vi "movearea.vi"(8 "error in (no error)":errorcluster, 11 "Input":string="y-") -> (0 "error out":errorcluster={"status"=TRUE, "code"=56, "source"="LabVIEWSMTPClient.lvlib:Send.vi:2280002<APPEND>\n\n<b>Complete call chain:</b>\r\n     LabVIEWSMTPClient.lvlib:Send.vi:2280002\r\n     Send Email using SMTP Client.vi:2070001\r\n     movearea.vi\r\n     parse and execute command.vi\r\n     TCPIP.Server v2.vi"}, 3 "Output":string="Approach area changed with 0 crashes ")   [LabVIEW 2014]
uses:
  <userlib>/Nanonis Prog Interface V5/Nanonis Prog Interface.lvlib
panel:
  out "num steps z":dbl=500.0
  out "testing?":bool
  out "status":string="approaching"
  in  "STMStatus":T1 {"Size (m)"."Height" format="%.2p"; "Size (m)"."Width" format="%.2p"; "Current (A)" format="%#_6p"; "Z position (m)" format="%#_6p"; "Center coordinates (m)"."Yc" format="%.2p"; "Center coordinates (m)"."Xc" format="%.2p"}
  out "size(s)":i32=1
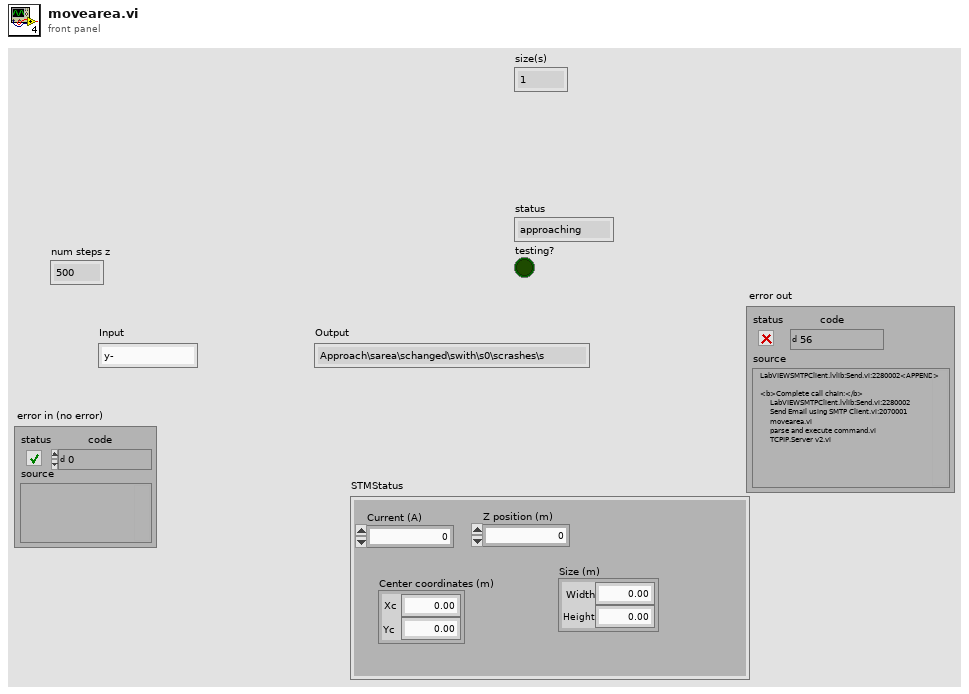
[diagram p1: front panel]
types:
  T1 = cluster{"Center coordinates (m)":cluster{"Xc":sgl, "Yc":sgl}, "Z position (m)":sgl, "Current (A)":sgl, "Size (m)":cluster{"Width":sgl, "Height":sgl}}
  T2 = enum8{"Group 1", "Group 2", "Group 3", "Group 4", "Group 5", "Group 6"}
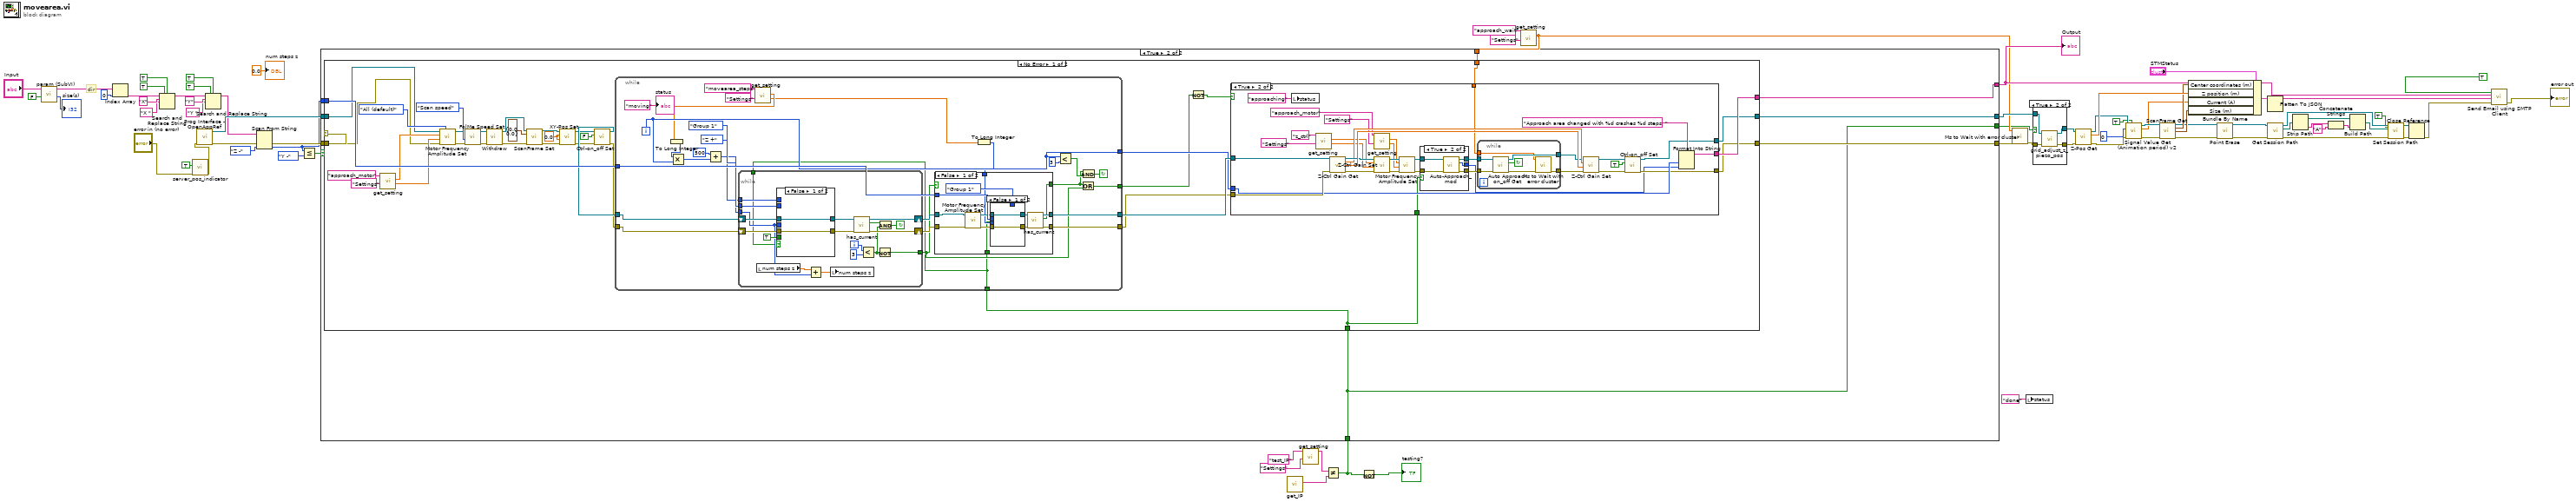
[diagram p0: block diagram]
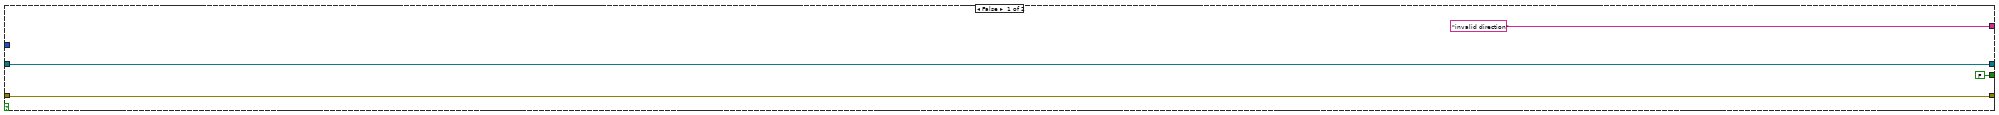
[diagram p3: hidden frame]
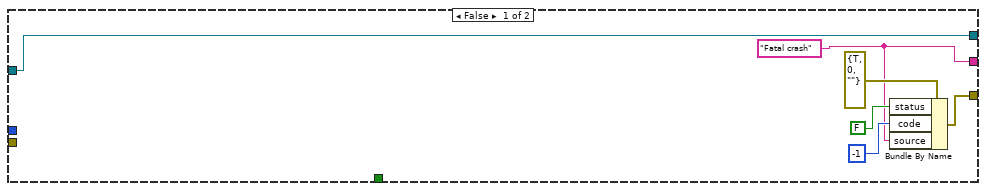
[diagram p4: hidden frame]
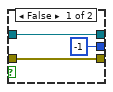
[diagram p5: hidden frame]
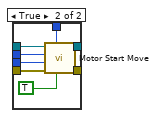
[diagram p6: hidden frame]
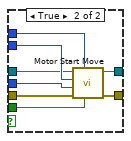
[diagram p8: hidden frame]
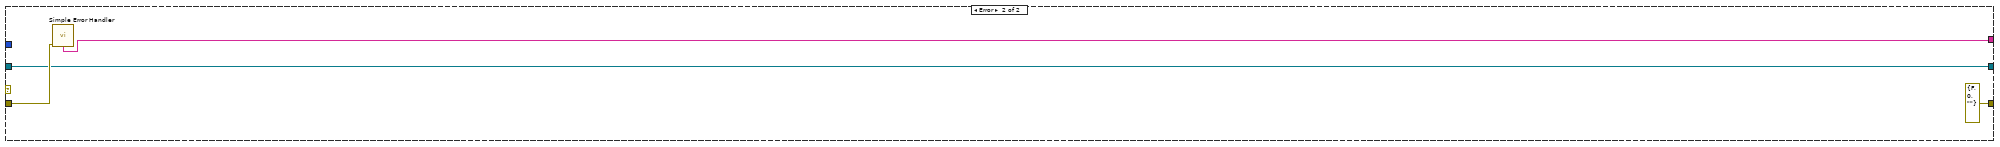
[diagram p9: hidden frame]
diagram:
  # "dir"
  n1 = call <userlib>:"param (SubVI).vi"("Numeric"=FALSE, "Input"="Input") -> ("num"=→"size(s)":i32, "Array"=w72:string[])  [unwired: 7 in, 1 out]
  n2 = Index Array(array=w72, index=0) -> (element=w63:string)
  n3 = Search and Replace String(replace all?=TRUE ("replace all? (F)"), case sensitive?=TRUE ("ignore case? (F)"), input string=w63, search string="X", replace string="X " ("replace string (\"\")")) -> (result string=w54:string)  [unwired: 3 in, 3 out]
  n4 = call "server_pos_indicator.vi"("reset"=TRUE, "error in"="error in (no error)") -> ("error out"=w23:errorcluster)  [unwired: 9 in]
  n5 = call <userlib>:"Prog Interface - OpenAppRef.vi"("Error in (no error)"=w23) -> ("Error out"=w69:errorcluster, "Application reference"=w73:refnum<vi>)  [unwired: 5 in]
  n6 = Search and Replace String(replace all?=TRUE ("replace all? (F)"), case sensitive?=TRUE ("ignore case? (F)"), input string=w54, search string="Y", replace string="Y " ("replace string (\"\")")) -> (result string=w53:string)  [unwired: 3 in, 3 out]
  n7 = Scan From String(input string=w53, error in=w69, default 1=enum16{"X +", "X -", "Y +", "Y -", "Z +", "Z -"}."Z -" ("Direction")) -> (error out=w68:errorcluster, output 1=w67:enum16{"X +", "X -", "Y +", "Y -", "Z +", "Z -"})  [unwired: 2 in, 2 out]
  n8 = Less Or Equal?(x=w67, y=enum16{"X +", "X -", "Y +", "Y -", "Z +", "Z -"}."Y -") -> (x <= y?=w65:bool)
  n9 = call "get_IP.vi"() -> ("IP address"=w39:string)  [unwired: 11 in]
  n10 = call "get_setting.vi"("section"="Settings", "key"="test_IP" ("IP Address")) -> ("value"=w20:string)  [unwired: 5 in, 4 out]
  n11 = Not Equal?(x=w20, y=w39) -> (x != y?=w37:bool)
  n12 = Not(x=w37) -> (.not. x?=→"testing?":bool)
  n13 = call "get_setting.vi"("section"="Settings", "key"="approach_wait") -> ("output 1"=w16:dbl)  [unwired: 5 in, 4 out]
  n14 = case shown="True" w65 {
    tunnel: w73 -> [w77 w87]
    tunnel: w67 -> [_ w86]
    tunnel: w68 -> [w79 w85]
    tunnel: [w79 w84] -> w28
    tunnel: ["invalid direction" ("message") w83] -> w35
    tunnel: [w77 w82] -> w27
    tunnel: w37 -> [_ w80]
    tunnel: w16 -> [_ w81]
    tunnel: [FALSE w80] -> w15
    frame False {
    }
    frame True {
      n15 = case shown="No Error" w85 {
        tunnel: w87 -> [w89 w259]
        tunnel: w86 -> [w110 _]
        tunnel: w85 -> [w88 w262]
        tunnel: [w97 errorcluster {"status"=FALSE, "code"=0, "source"=""} ("error out")] -> w84
        tunnel: [w102 w261] -> w83
        tunnel: [w96 w259] -> w82
        tunnel: w80 -> [w90 _]
        tunnel: w81 -> [w91 _]
        frame No Error {
          w116 = sgl 0.0 ("X (m)")
          n16 = call "get_setting.vi"("section"="Settings", "key"="approach_motor") -> ("output 2"=w92:dbl, "output 1"=w93:dbl)  [unwired: 5 in, 3 out]
          n17 = call <userlib>:"Motor Frequency Amplitude Set.vi"("Axis (All)"=enum16{"All (default)", "X", "Y", "Z"}."All (default)", "Error in (no error)"=w88, "Amplitude (V) (NaN=no change)"=w92, "Frequency (Hz) (NaN=no change)"=w93, "Application ref in"=w89) -> ("Error out"=w109:errorcluster, "Application ref out"=w111:refnum<vi>)  [unwired: 5 in]
          n18 = call <userlib>:"FolMe Speed Set.vi"("error in (no error)"=w109, "Speed Setting (Custom)"=enum32{"Scan speed", "Custom speed"}."Scan speed", "Application ref in"=w111) -> ("error out"=w113:errorcluster, "Application ref out"=w114:refnum<vi>)  [unwired: 5 in]
          n19 = call <userlib>:"Withdraw.vi"("Error in (no error)"=w113, "Application ref in"=w114) -> ("Error out"=w120:errorcluster, "Application ref out"=w121:refnum<vi>)  [unwired: 8 in]
          n20 = call <userlib>:"ScanFrame Set.vi"("Application ref in"=w121, "Center coordinates (m)"=cluster{"Xc":sgl, "Yc":sgl} {"Xc"=0.0, "Yc"=0.0}, "error in (no error)"=w120) -> ("Application ref out"=w117:refnum<vi>, "error out"=w118:errorcluster)  [unwired: 11 in]
          n21 = call <userlib>:"XY-Pos Set.vi"("error in (no error)"=w118, "Y (m)"=w116, "X (m)"=w116, "Application ref in"=w117) -> ("error out"=w103:errorcluster, "Application ref out"=w104:refnum<vi>)  [unwired: 4 in]
          n22 = call <userlib>:"Ctrl-on_off Set.vi"("error in (no error)"=w103, "Z Controller ON/OFF"=FALSE, "Application ref in"=w104) -> ("error out"=w105:errorcluster, "Application ref out"=w106:refnum<vi>)  [unwired: 7 in]
          n23 = while {
            tunnel: w110 -> [w203]
            tunnel: [w194] -> w108
            tunnel: [w193] -> w107
            tunnel: w106 -> [w192]
            tunnel: w105 -> [w191]
            tunnel: [w190] -> w101
            tunnel: [w185] -> w100
            tunnel: w90 -> [w177]
            i -> [w190]
            stop <- w196 continue-if-true
            n24 = call "get_setting.vi"("section"="Settings", "key"="movearea_steps") -> ("output 2"=w179:dbl, "output 1"=w181:dbl)  [unwired: 5 in, 3 out]
            n25 = To Long Integer(number=w181) -> (32bit integer=w180:i32)
            n26 = Multiply(x=w180, y=w190) -> (x*y=w199:i32)
            n27 = Add(x=u16 500 ("Number of steps"), y=w199) -> (x+y=w200:i32)
            n28 = while {
              tunnel: enum16{"X +", "X -", "Y +", "Y -", "Z +", "Z -"}."Z +" ("Direction") -> [w248]
              tunnel: T2."Group 1" ("Group") -> [w246]
              tunnel: w200 -> [w232]
              shift-right: [w243] -> w187
              shift-left: w192 -> [w245]
              shift-right: [w240] -> w186
              shift-left: w191 -> [w244]
              tunnel: [w234] -> w184
              tunnel: w177 -> [w230]
              i -> [w238]
              stop <- w236 continue-if-true
              n29 = local read "num steps z"() -> (w233:dbl)
              n30 = case shown="False" w230 {
                tunnel: w248 -> [_ w258]
                tunnel: TRUE ("Wait until finished? (F)") -> [_ w257]
                tunnel: w246 -> [_ w256]
                tunnel: w245 -> [w250 w255]
                tunnel: w244 -> [w249 w254]
                tunnel: [w250 w253] -> w242
                tunnel: [w249 w252] -> w241
                tunnel: w232 -> [_ w251]
                frame False {
                }
                frame True {
                  n31 = call <userlib>:"Motor Start Move.vi"("Wait until finished? (F)"=w257, "Group"=w256, "Error in (no error)"=w254, "Number of steps"=w251, "Direction"=w258, "Application ref in"=w255) -> ("Error out"=w252:errorcluster, "Application ref out"=w253:refnum<vi>)  [unwired: 3 in]
                }
              }
              n32 = Add(x=w233, y=w232) -> (x+y=w231:dbl)
              n33 = local write "num steps z"(w231) -> ()
              n34 = call "has_current.vi"("error in (no error)"=w241, "Application in"=w242) -> ("error out"=w240:errorcluster, "Boolean"=w237:bool, "Application out"=w243:refnum<vi>)  [unwired: 7 in]
              n35 = Less?(x=w238, y=3) -> (x < y?=w235:bool)
              n36 = Not(x=w235) -> (.not. x?=w234:bool)
              n37 = And(x=w237, y=w235) -> (x .and. y?=w236:bool)
            }
            n38 = To Long Integer(number=w179) -> (32bit integer=w178:i32)
            n39 = case shown="False" w184 {
              selector: w184 -> [_ w227]
              tunnel: w203 -> [w216 _]
              tunnel: [w212 w228] -> w194
              tunnel: [w211 w229] -> w193
              tunnel: [w210 w227] -> w189
              tunnel: w187 -> [w207 w228]
              tunnel: w186 -> [w206 w229]
              tunnel: w178 -> [w205 _]
              tunnel: w177 -> [w204 _]
              frame False {
                n40 = call <userlib>:"Motor Frequency Amplitude Set.vi"("Error in (no error)"=w206, "Application ref in"=w207) -> ("Error out"=w208:errorcluster, "Application ref out"=w209:refnum<vi>)  [unwired: 8 in]
                n41 = case shown="False" w204 {
                  tunnel: w216 -> [_ w226]
                  tunnel: T2."Group 1" ("Group") -> [_ w224]
                  tunnel: [w218 w223] -> w214
                  tunnel: [w217 w222] -> w213
                  tunnel: w209 -> [w218 w221]
                  tunnel: w208 -> [w217 w220]
                  tunnel: w205 -> [_ w219]
                  frame False {
                  }
                  frame True {
                    n42 = call <userlib>:"Motor Start Move.vi"("Wait until finished? (F)"=TRUE, "Group"=w224, "Error in (no error)"=w220, "Number of steps"=w219, "Direction"=w226, "Application ref in"=w221) -> ("Error out"=w222:errorcluster, "Application ref out"=w223:refnum<vi>)  [unwired: 3 in]
                  }
                }
                n43 = call "has_current.vi"("error in (no error)"=w213, "Application in"=w214) -> ("error out"=w211:errorcluster, "Boolean"=w210:bool, "Application out"=w212:refnum<vi>)  [unwired: 7 in]
              }
              frame True {
              }
            }
            n44 = Less?(x=w190, y=3) -> (x < y?=w195:bool)
            n45 = Or(x=w189, y=w184) -> (x .or. y?=w185:bool)
            n46 = And(x=w189, y=w195) -> (x .and. y?=w196:bool)
            "status" <- "moving"
          }
          n47 = Not(x=w100) -> (.not. x?=w99:bool)
          n48 = case shown="True" w99 {
            tunnel: w108 -> [w122 w161]
            tunnel: w107 -> [_ w155]
            tunnel: [w124 w148] -> w102
            tunnel: w101 -> [_ w147]
            tunnel: [w123 w129] -> w97
            tunnel: [w122 w130] -> w96
            tunnel: w90 -> [_ w131]
            tunnel: w91 -> [_ w132]
            frame False {
              w124 = "Fatal crash"
              n49 = Bundle By Name(cluster=errorcluster {"status"=TRUE, "code"=0, "source"=""} ("error out"), "status"=FALSE, "code"=-1, "source"=w124) -> (w123:errorcluster)
            }
            frame True {
              n50 = local write "status"("approaching" ("status")) -> ()
              n51 = call "get_setting.vi"("section"="Settings", "key"="z_ctrl" ("IP Address")) -> ("output 2"=w133:dbl, "output 1"=w134:dbl)  [unwired: 5 in, 3 out]
              n52 = call <userlib>:"Z-Ctrl Gain Get.vi"("Application ref in"=w161, "error in (no error)"=w155) -> ("Application ref out"=w159:refnum<vi>, "P-gain"=w158:sgl, "Time constant (s)"=w160:sgl, "error out"=w154:errorcluster)  [unwired: 9 in, 1 out]
              n53 = call "get_setting.vi"("section"="Settings", "key"="approach_motor" ("IP Address")) -> ("output 2"=w137:dbl, "output 1"=w138:dbl)  [unwired: 5 in, 3 out]
              n54 = call <userlib>:"Z-Ctrl Gain Set.vi"("error in (no error)"=w154, "Time constant (s)"=w133, "P-gain"=w134, "Application ref in"=w159) -> ("error out"=w143:errorcluster, "Application ref out"=w144:refnum<vi>)  [unwired: 5 in]
              n55 = call <userlib>:"Motor Frequency Amplitude Set.vi"("Error in (no error)"=w143, "Amplitude (V) (NaN=no change)"=w137, "Frequency (Hz) (NaN=no change)"=w138, "Application ref in"=w144) -> ("Error out"=w141:errorcluster, "Application ref out"=w142:refnum<vi>)  [unwired: 6 in]
              n56 = case shown="True" w131 {
                tunnel: [w163 w169] -> w157
                tunnel: [w164 w168] -> w153
                tunnel: w142 -> [w163 w167]
                tunnel: w141 -> [w164 w166]
                tunnel: [-1 ("steps taken") w165] -> w128
                frame False {
                }
                frame True {
                  n57 = call "Auto-Approach_mod.vi"("Error in"=w166, "Application reference"=w167) -> ("error out"=w168:errorcluster, "steps taken"=w165:i32, "Application ref out"=w169:refnum<vi>)  [unwired: 4 in, 1 out]
                }
              }
              n58 = while {
                tunnel: w157 -> [w175]
                tunnel: [w174] -> w156
                tunnel: w153 -> [w173]
                tunnel: [w172] -> w152
                tunnel: w132 -> [w171]
                stop <- w170 continue-if-true
                n59 = call <userlib>:"Auto Approach on_off Get.vi"("Error in (no error)"=w173, "Application ref in"=w175) -> ("Error out"=w176:errorcluster, "Auto approach on/off status"=w170:bool, "Application ref out"=w174:refnum<vi>)  [unwired: 5 in]
                n60 = call <userlib>:"Ms to Wait with error cluster.vi"("error in (no error)"=w176, "milliseconds to wait"=w171) -> ("error out"=w172:errorcluster)  [unwired: 4 in, 1 out]
              }
              n61 = call <userlib>:"Z-Ctrl Gain Set.vi"("error in (no error)"=w152, "Time constant (s)"=w160, "P-gain"=w158, "Application ref in"=w156) -> ("error out"=w149:errorcluster, "Application ref out"=w151:refnum<vi>)  [unwired: 5 in]
              n62 = call <userlib>:"Ctrl-on_off Set.vi"("error in (no error)"=w149, "Z Controller ON/OFF"=TRUE, "Application ref in"=w151) -> ("error out"=w129:errorcluster, "Application ref out"=w130:refnum<vi>)  [unwired: 7 in]
              n63 = Format Into String(format string="Approach area changed with %d crashes %d steps  " ("initial string"), w147, w128) -> (resulting string=w148:string)  [unwired: 2 in, 1 out]
            }
          }
        }
        frame Error {
          n64 = call <vilib>:"Simple Error Handler.vi"("error in (no error)"=w262) -> ("message"=w261:string)  [unwired: 4 in, 4 out]
        }
      }
    }
  }
  "Output" <- w35
  n65 = call <userlib>:"Ms to Wait with error cluster.vi"("error in (no error)"=w28, "milliseconds to wait"=w16) -> ("error out"=w30:errorcluster)  [unwired: 4 in, 1 out]
  n66 = local write "status"("done" ("status")) -> ()
  n67 = case shown="True" w15 {
    tunnel: w30 -> [w263 w268]
    tunnel: [w263 w267] -> w29
    tunnel: w27 -> [w264 w266]
    tunnel: [w264 w265] -> w26
    frame False {
    }
    frame True {
      n68 = call "grid_adjust_z_piezo_pos.vi"("Error in (no error)"=w268, "Application ref in"=w266) -> ("Error out"=w267:errorcluster, "Application ref out"=w265:refnum<vi>)  [unwired: 8 in]
    }
  }
  n69 = call <userlib>:"Z-Pos Get.vi"("error in (no error)"=w29, "Application ref in"=w26) -> ("error out"=w44:errorcluster, "Z position (m)"=w50:sgl, "Application ref out"=w47:refnum<vi>)  [unwired: 7 in]
  n70 = call <userlib>:"Signal Value Get (Animation period) v2.vi"("Wait for newest data (F=False)"=TRUE, "error in (no error)"=w44, "Signal index (0-79)"=i8 0, "Application ref in"=w47) -> ("error out"=w45:errorcluster, "Signal value"=w42:sgl, "Application ref out"=w46:refnum<vi>)  [unwired: 4 in]
  n71 = call <userlib>:"ScanFrame Get.vi"("Application ref in"=w46, "error in (no error)"=w45) -> ("Application ref out"=w31:refnum<vi>, "Center coordinates (m)"=w49:cluster{"Xc":sgl, "Yc":sgl}, "Size (m)"=w48:cluster{"Width":sgl, "Height":sgl}, "error out"=w32:errorcluster)  [unwired: 9 in, 1 out]
  n72 = Bundle By Name(cluster="STMStatus", "Center coordinates (m)"=w49, "Z position (m)"=w50, "Current (A)"=w42, "Size (m)"=w48) -> (w51:T1)
  n73 = call <userlib>:"Point Erase.vi"("Application ref in"=w31, "error in (no error)"=w32) -> ("Application ref out"=w13:refnum<vi>, "error out"=w8:errorcluster)  [unwired: 12 in]
  n74 = Flatten To JSON(anything=w51) -> (JSON string=w34:string)  [unwired: 2 in, 1 out]
  n75 = call <userlib>:"Get Session Path.vi"("error in (no error)"=w8, "Application ref in"=w13) -> ("error out"=w10:errorcluster, "Session path"=w4:path, "Application ref out"=w12:refnum<vi>)  [unwired: 7 in]
  n76 = Strip Path(path=w4) -> (stripped path=w5:path, name=w2:string)
  n77 = Concatenate Strings(w2, "A" ("string")) -> (w3:string)
  n78 = Build Path(base path=w5, name or relative path=w3) -> (appended path=w6:path)
  n79 = call <userlib>:"Set Session Path.vi"("Save settings to previous? (False)"=TRUE, "error in (no error)"=w10, "Session Folder"=w6, "Application ref in"=w12) -> ("error out"=w9:errorcluster, "Application ref out"=w11:refnum<vi>)  [unwired: 6 in]
  n80 = Close Reference(reference=w11, error in (no error)=w9) -> (error out=w33:errorcluster)
  n81 = call "Send Email using SMTP Client.vi"("map?"=TRUE, "error in (no error)"=w33, "Message"=w34, "subject"=w35) -> ("error out"=→"error out":errorcluster)  [unwired: 7 in]
  "num steps z" <- 0.0 ("num steps z")
